vi "Template Test.vi"(0 "Limits File Path":path, 5 "Results File Path":path, 11 "error in":errorcluster) -> (15 "error out":errorcluster)   [LabVIEW 2024]
doc: "Template test"
uses:
  <vilib>/addons/_JKI Toolkits/State Machine/_JKI_lib_State_Machine.llb/Select State(s)_err__jki_lib_state_machine.vi
  <vilib>/addons/_JKI Toolkits/State Machine/_JKI_lib_State_Machine.llb/Periodic Trigger__ogtk__JKI-SM__jki_lib_state_machine.vi
  <userlib>/_OpenG.lib/file/file.llb/Strip Path Extension - String__ogtk.vi
  <vilib>/Utility/file.llb/Read Delimited Spreadsheet (string).vi
  <vilib>/Utility/file.llb/Write Delimited Spreadsheet (string).vi
  <userlib>/_OpenG.lib/file/file.llb/openg_file.lvlib
  <userlib>/_OpenG.lib/appcontrol/appcontrol.llb/openg_application_control.lvlib
  <userlib>/_OpenG.lib/time/time.llb/openg_time.lvlib
panel:
  out "Voltage Results Data":string[](array[string])
  in  "Exit":bool
  # "LED Test VI"
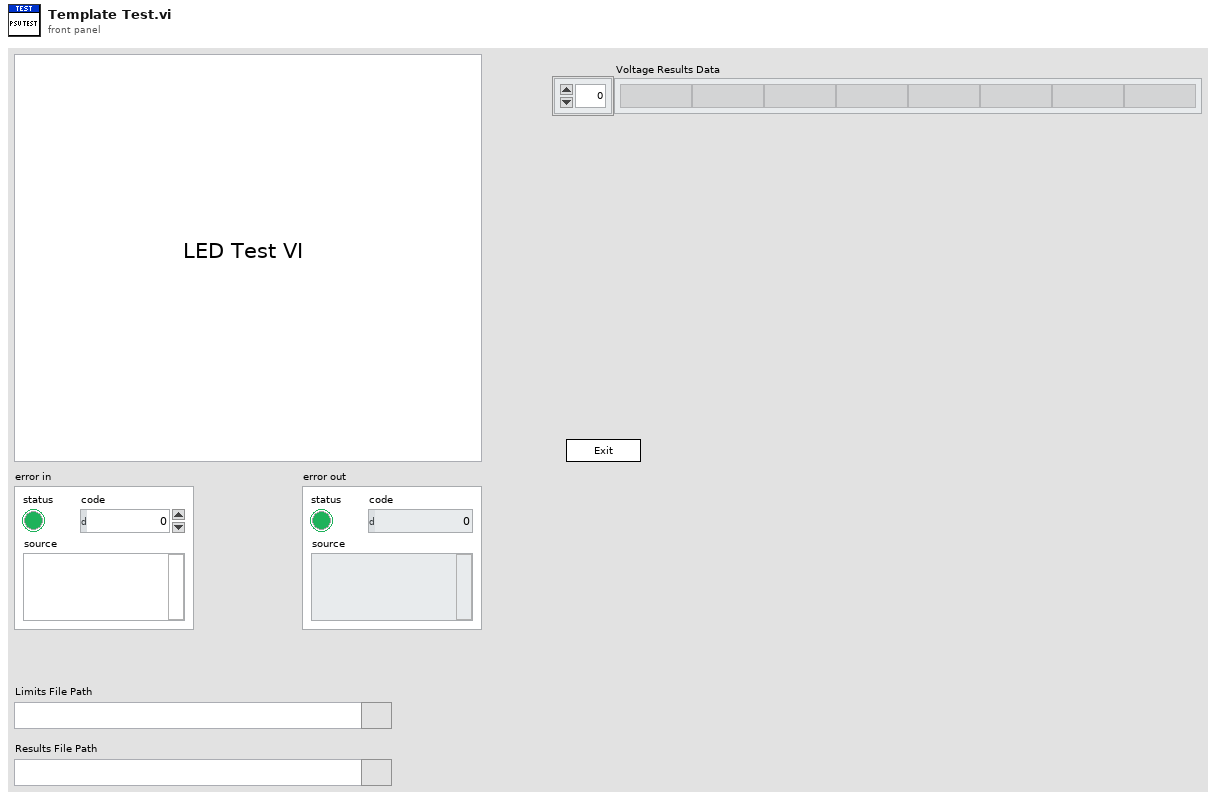
[diagram p1: front panel]
types:
  T1 = enum32{"Invalid", "Standard", "Closed", "Hidden", "Minimized", "Maximized"}
  T2 = enum32{"invalid app kind", "Development System", "Run Time System", "Student Edition", "Embedded LabVIEW", "Evaluation", "Custom"}
  T3 = cluster{"Core":cluster{"Current VI Reference":refnum<vi>, "Close Panel on Exit?":bool}, "Limits File Path":path, "Test Limits":string[][], "Results Data Array":string[][], "Results File Path":path, "Voltage":dbl}
  T4 = cluster{"Current VI Reference":refnum<vi>, "Close Panel on Exit?":bool}
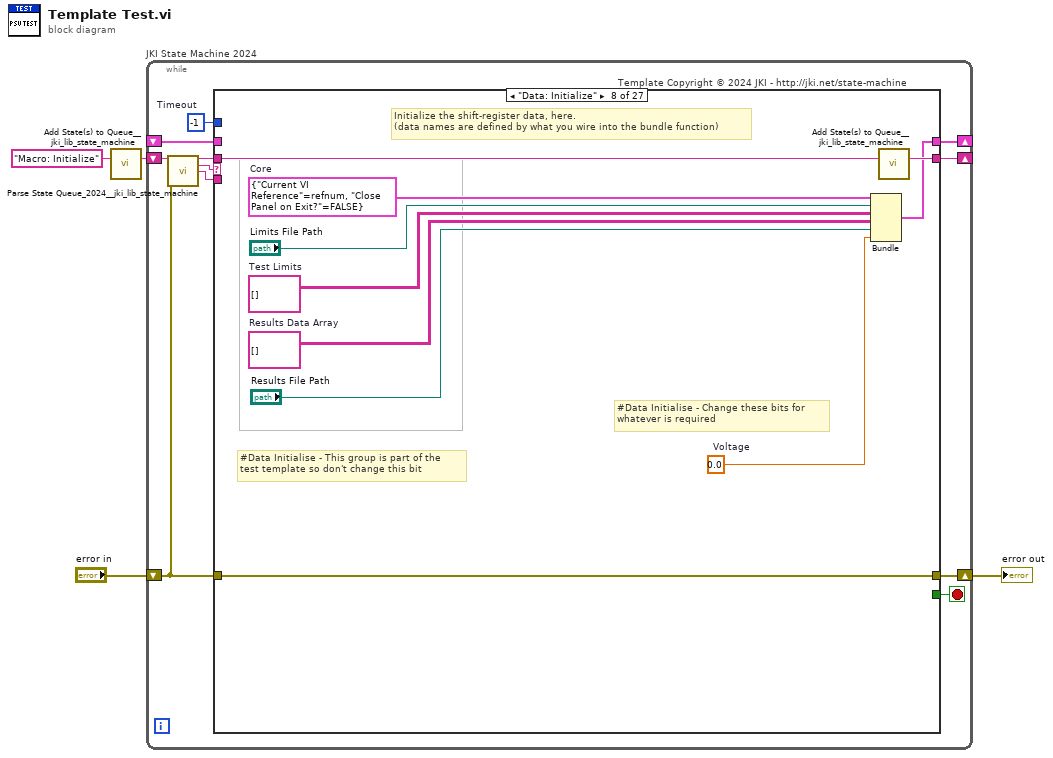
[diagram p0: block diagram]
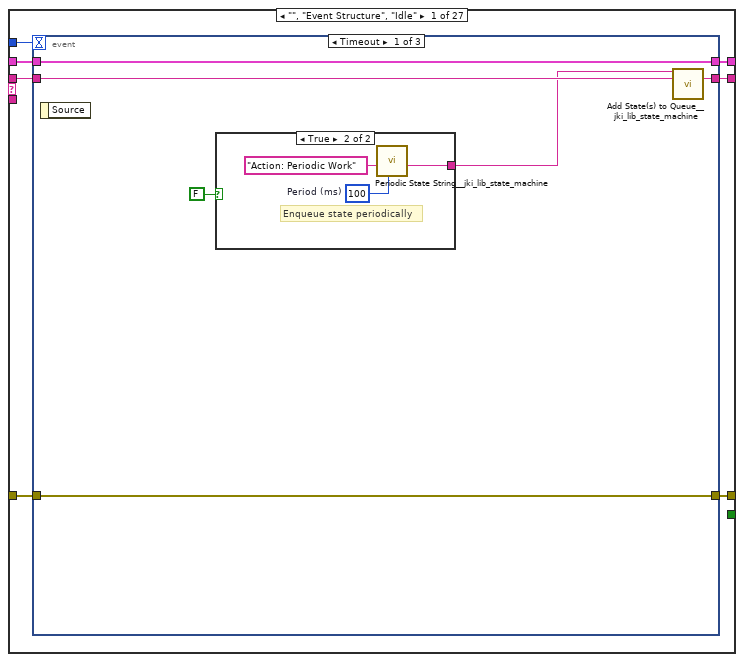
[diagram p2: hidden frame]
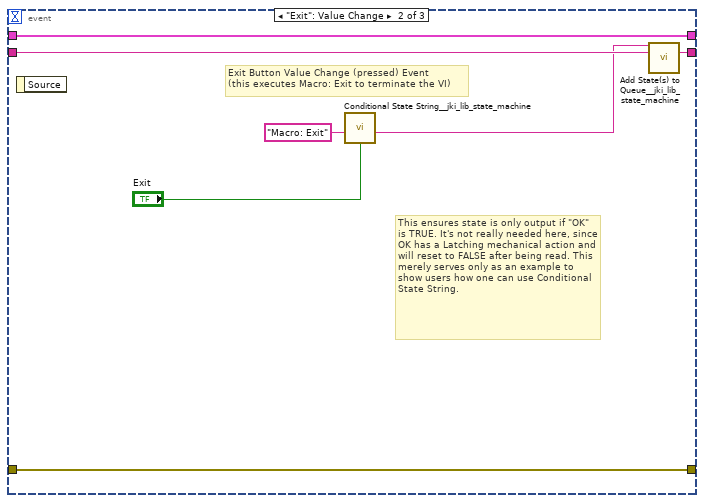
[diagram p4: hidden frame]
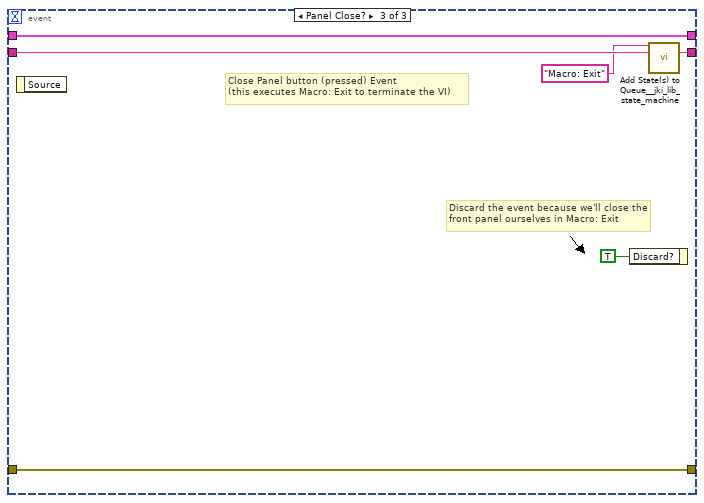
[diagram p5: hidden frame]
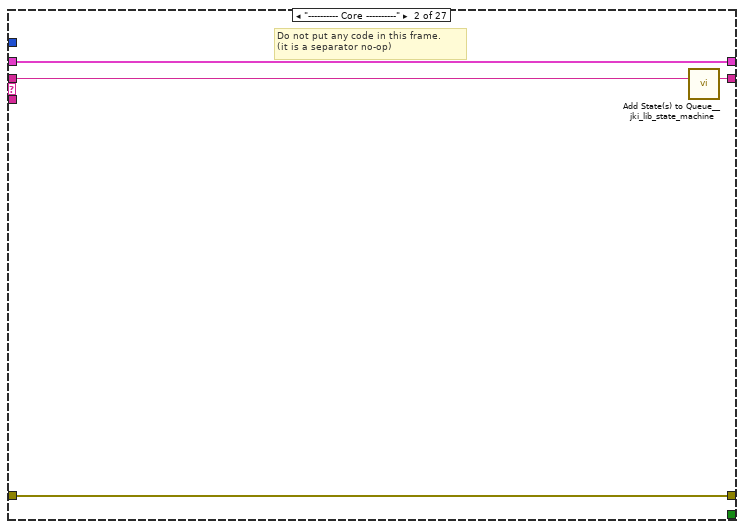
[diagram p6: hidden frame]
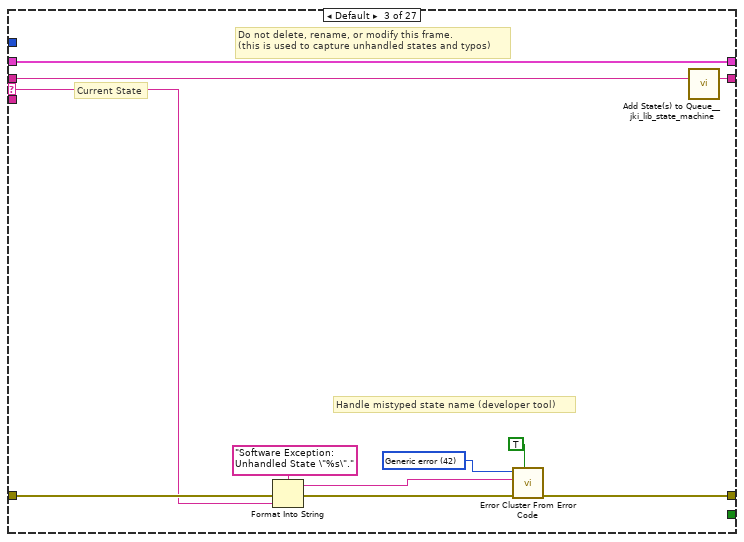
[diagram p7: hidden frame]
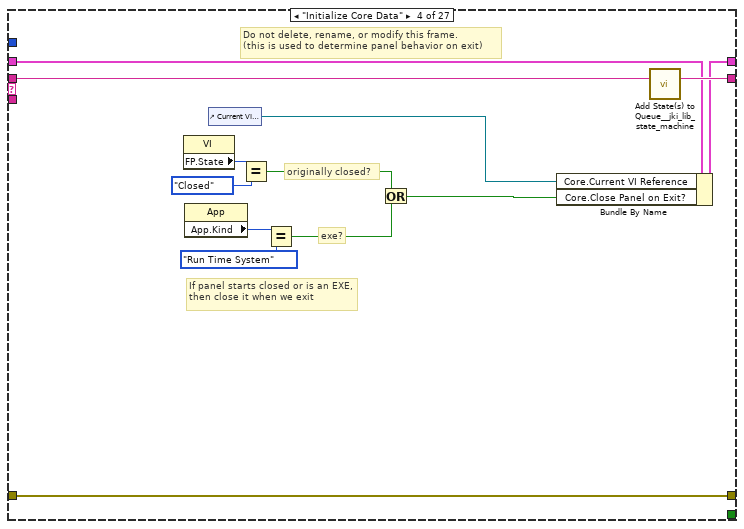
[diagram p8: hidden frame]
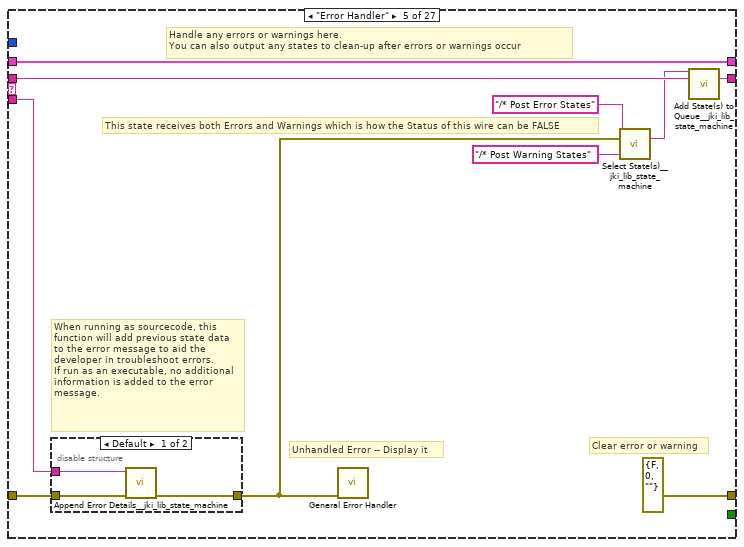
[diagram p9: hidden frame]
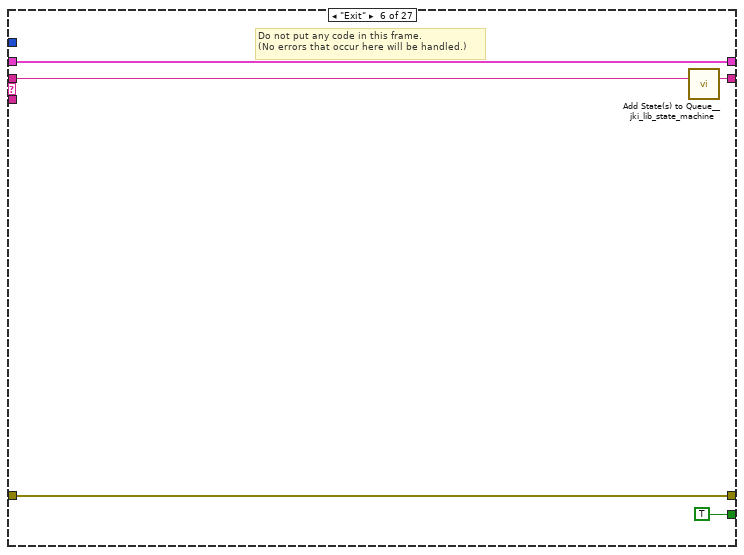
[diagram p11: hidden frame]
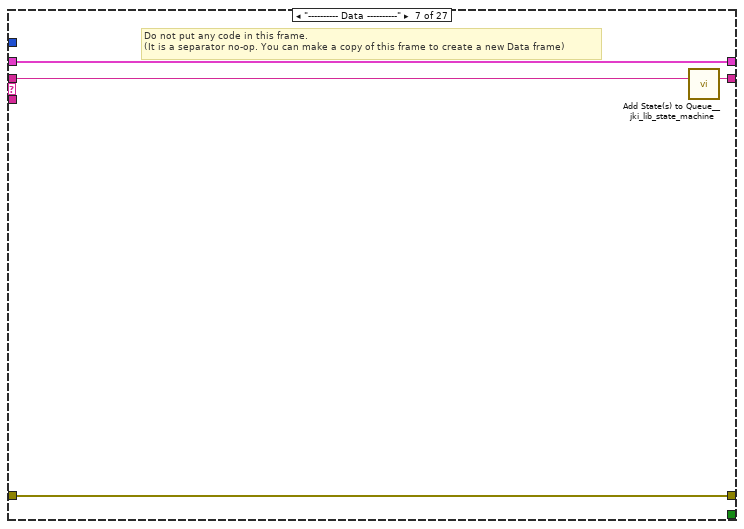
[diagram p12: hidden frame]
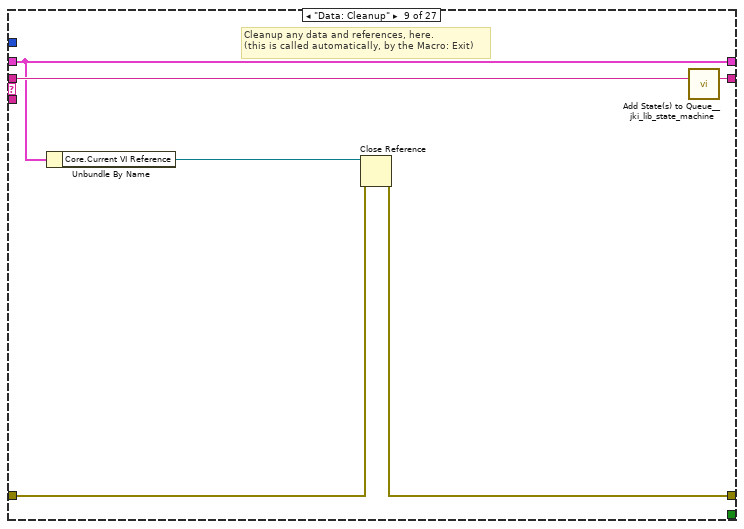
[diagram p13: hidden frame]
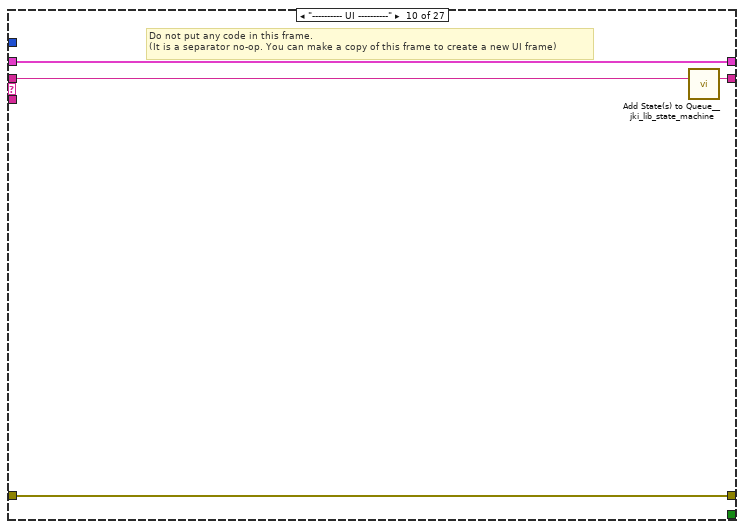
[diagram p14: hidden frame]
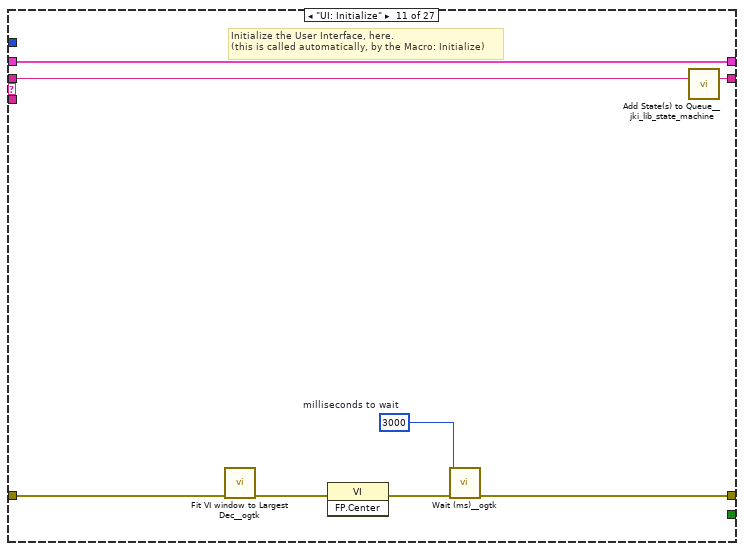
[diagram p15: hidden frame]
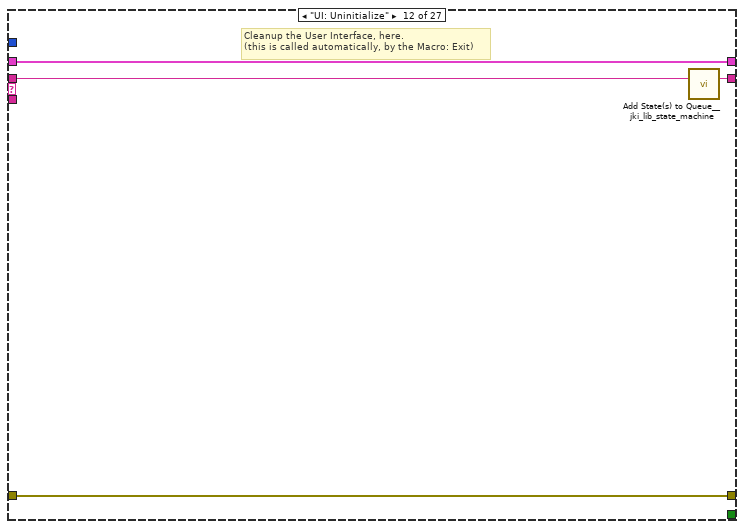
[diagram p16: hidden frame]
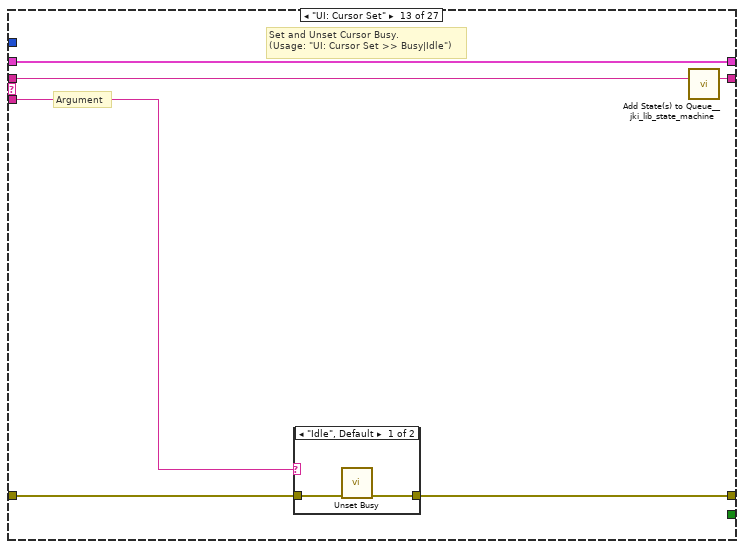
[diagram p17: hidden frame]
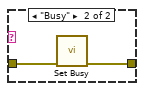
[diagram p18: hidden frame]
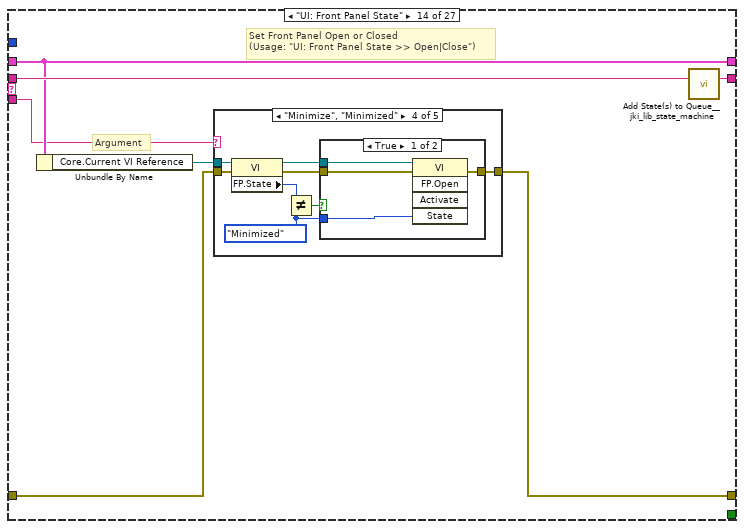
[diagram p19: hidden frame]
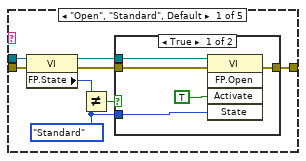
[diagram p20: hidden frame]
diagram:
  n1 = call <vilib>:"Add State(s) to Queue__jki_lib_state_machine.vi"("State(s) in (\"\")"="Macro: Initialize") -> ("States Out"=w4:string)  [unwired: 14 in]
  n2 = while "JKI State Machine 2024" {
    shift-right: [w8] -> _
    shift-left: _ -> [w7]
    shift-right: [w11] -> w1
    shift-left: "error in" -> [w5]
    shift-right: [w10] -> _
    shift-left: w4 -> [w12]
    stop <- w9 stop-if-true
    w6 = -1  # Timeout
    # "Template Copyright © 2024 JKI - http://jki.net/state-machine"
    n3 = call <vilib>:"Parse State Queue_2024__jki_lib_state_machine.vi"("State Queue"=w12, "Error In (no error)"=w5) -> ("Remaining States"=w14:string, "Current State"=w15:string, "Arguments"=w13:string)  [unwired: 11 in]
    n4 = case shown="\"Data: Initialize\"" w15 {
      selector: w15 -> [_ _ w49 _ _ _ _ _ _ _ _ _ _ _ _ _ _ _ _ _ _ _ _ _ _ _ _]
      tunnel: w14 -> [w22 w48 w53 w72 w82 w91 w95 w105 w111 w115 w123 w127 w133 w144 w213 w218 w222 w231 w235 w248 w265 w269 w278 w282 w286 w292 w296]
      tunnel: w13 -> [_ _ _ _ w77 _ _ _ _ _ _ _ w128 w138 _ _ _ _ _ _ _ _ _ _ _ _ _]
      tunnel: w7 -> [w20 w45 w51 w65 w79 w89 w92 _ w106 w112 w121 w125 w131 w140 w210 w215 w219 w229 w232 w238 w257 w266 w274 w279 w283 w289 w293]
      tunnel: [w19 w46 w55 w69 errorcluster {"status"=FALSE, "code"=0, "source"=""} ("error out") w88 w93 w102 w107 w113 w119 w124 w129 w141 w211 w216 w220 w226 w233 w244 w262 w267 w276 w280 w284 w290 w294] -> w11
      tunnel: w5 -> [w16 w46 w54 w69 w78 w88 w93 w102 w108 w113 w120 w124 w130 w142 w211 w216 w220 w226 w233 w243 w261 w267 w275 w280 w284 w290 w294]
      tunnel: [w21 w47 w52 w71 w81 w90 w94 w104 w110 w114 w122 w126 w132 w143 w212 w217 w221 w230 w234 w247 w264 w268 w277 w281 w285 w291 w295] -> w10
      tunnel: [_ _ _ _ _ TRUE _ _ _ _ _ _ _ _ _ _ _ _ _ _ _ _ _ _ _ _ _] -> w9
      tunnel: [w18 w45 w51 w70 w79 w89 w92 w103 w106 w112 w121 w125 w131 w140 w210 w215 w219 w229 w232 w237 w256 w266 w274 w279 w283 w288 w293] -> w8
      tunnel: w6 -> [w17 _ _ _ _ _ _ _ _ _ _ _ _ _ _ _ _ _ _ _ _ _ _ _ _ _ _]
      frame "", "Event Structure", "Idle" {
        n5 = event shown="[0] Timeout" {
          selector: _ -> [_ _ _]
          dyn-events: _ -> [_ _ _]
          timeout: w17 -> [_ _ _]
          tunnel: w22 -> [w28 w38 w44]
          tunnel: [w27 w37 w43] -> w21
          tunnel: w20 -> [w25 w35 w41]
          tunnel: [w26 w36 w42] -> w19
          tunnel: w16 -> [w26 w36 w42]
          tunnel: [w25 w35 w41] -> w18
          event Timeout {
            n6 = event-data() -> ()  [unwired: 1 in, 1 out]
            n7 = case shown="True" FALSE {
              tunnel: [_ w31] -> w24
              frame False {
              }
              frame True {
                w29 = u32 100  # Period (ms)
                # "Enqueue state periodically"
                n8 = call <vilib>:"Periodic State String__jki_lib_state_machine.vi"("Period (ms)"=w29, "State"="Action: Periodic Work") -> ("State Out"=w31:string)  [unwired: 9 in]
              }
            }
            n9 = call <vilib>:"Add State(s) to Queue__jki_lib_state_machine.vi"("State(s) in Front (\"\")"=w24, "State(s) in (\"\")"=w28) -> ("States Out"=w27:string)  [unwired: 13 in]
          }
          event "Exit": Value Change {
            # "This ensures state is only output if \"OK\" is TRUE. It's not really needed here, since OK has a Latching mechanical action and will reset to FALSE after being read. This merely serves only as an example to show users how one can use Conditional State String."
            # "Exit Button Value Change (pressed) Event\n(this executes Macro: Exit to terminate the VI)"
            n10 = event-data() -> ()  [unwired: 1 in, 1 out]
            n11 = call <vilib>:"Conditional State String__jki_lib_state_machine.vi"("Do State(s)?"="Exit", "State"="Macro: Exit") -> ("State Out"=w32:string)  [unwired: 7 in]
            n12 = call <vilib>:"Add State(s) to Queue__jki_lib_state_machine.vi"("State(s) in Front (\"\")"=w32, "State(s) in (\"\")"=w38) -> ("States Out"=w37:string)  [unwired: 13 in]
          }
          event Panel Close? {
            # "Discard the event because we'll close the front panel ourselves in Macro: Exit"
            # "Close Panel button (pressed) Event\n(this executes Macro: Exit to terminate the VI)"
            n13 = event-data() -> ()  [unwired: 1 in, 1 out]
            n14 = event-data("Discard?"=TRUE) -> ()  [unwired: 1 in, 1 out]
            n15 = call <vilib>:"Add State(s) to Queue__jki_lib_state_machine.vi"("State(s) in Front (\"\")"="Macro: Exit", "State(s) in (\"\")"=w44) -> ("States Out"=w43:string)  [unwired: 13 in]
          }
        }
      }
      frame "---------- Core ----------" {
        # "Do not put any code in this frame.\n(it is a separator no-op)"
        n16 = call <vilib>:"Add State(s) to Queue__jki_lib_state_machine.vi"("State(s) in (\"\")"=w48) -> ("States Out"=w47:string)  [unwired: 14 in]
      }
      frame Default {
        w58 = 42 items=["No error", "Argument error", "Memory is full", "Out of zone", "End of file", "File already open", "Generic file I/O error", "File not found", "File permission error", "Disk is full", "Duplicate path", "Too many files open", "System feature not enabled", "Resource file not found", "Cannot add resource", "Resource not found", "Image not found", "Image memory error", "Pen does not exist", "Config type invalid", "Config token not found", "Config parse error", "Config memory error", "Bad external code format", "Bad external code offset", "External code not present", "Null window", "Destroy window error", "Null menu", "Print aborted", "Bad print record", "Print driver error", "Windows error during printing", "Memory error during printing", "Print dialog error", "Generic print error", "Invalid device refnum", "Device not found", "Device parameter error", "Device unit error", "Cannot open device", "Device call aborted", "Generic error", "Cancelled by user", "Object ID too low", "Object ID too high", "Object not in heap", "Unknown heap", "Unknown object (invalid DefProc)", "Unknown object (DefProc not in table)", "Message out of range", "Invalid (null) method", "Unknown message", "Manager call not supported", "Bad address", "Network operation in progress", "Network operation timed out", "Connection is busy", "Network attribute not supported", "Network error", "Address in use", "System out of memory", "Connection aborted", "Connection refused", "Not connected", "Already connected", "Connection closed", "Initialization error (interapplication manager)", "Bad occurrence", "Wait on unbound occurrence handler", "Occurrence queue overflow", "Datalog type conflict", "Unused", "Unrecognized type (interapplication manager)", "Memory corrupt", "Failed to make temporary DLL", "Old CIN version", "Drag socket not found", "Failed to load drop-object", "Failed to register OLE object", "Failed to release OLE object", "Format specifier type mismatch", "Unknown format specifier", "Too few format specifiers", "Too many format specifiers", "Scan failed", "Newer CIN version", "Error converting to variant", "Runtime menu error", "Password tampered", "Variant attribute not found", "Incompatible variant data type", "Event data is not available", "Event Store is not present", "Occurrence is not found", "Event Queue is not created", "Event info is not available", "Refnum passed is NULL", "Error retrieving Class GUID", "Error retrieving CoClass GUID", "Error retrieving TypeLib GUID.", "Bad built application magic bytes.", "Specific driver is different from the specific driver associated with the Logical Name.", "There is no session opened to the class driver.", "Max Error", "MAX - Error with config objects", "MAX - Error loading configuration", "MAX - Group not supported"]
        # "Current State"
        # "Do not delete, rename, or modify this frame.\n(this is used to capture unhandled states and typos)"
        # "Handle mistyped state name (developer tool)"
        n17 = Format Into String(format string="Software Exception: Unhandled State \"%s\"." ("message"), error in=w54, w49) -> (resulting string=w57:string, error out=w56:errorcluster)  [unwired: 1 in]
        n18 = call <vilib>:"Error Cluster From Error Code.vi"("show call chain? (False)"=TRUE, "error in (no error)"=w56, "error message (\"\")"=w57, "error code (0)"=w58) -> ("error out"=w55:errorcluster)  [unwired: 5 in]
        n19 = call <vilib>:"Add State(s) to Queue__jki_lib_state_machine.vi"("State(s) in (\"\")"=w53) -> ("States Out"=w52:string)  [unwired: 14 in]
      }
      frame "Initialize Core Data" {
        # "Do not delete, rename, or modify this frame.\n(this is used to determine panel behavior on exit)"
        # "originally closed?"
        # "exe?"
        # "If panel starts closed or is an EXE, then close it when we exit"
        n20 = property class="VI"() -> ("FP.State"=w62:T1)  [unwired: 2 in, 2 out]
        n21 = property class="App"() -> ("App.Kind"=w68:T2)  [unwired: 2 in, 2 out]
        n22 = control-ref of="Current VI Reference"() -> (w63:refnum<vi>)
        n23 = Equal?(x=w62, y=T1."Closed" ("Front Panel Window:State")) -> (x = y?=w60:bool)
        n24 = Equal?(x=w68, y=T2."Run Time System" ("Application:Kind")) -> (x = y?=w66:bool)
        n25 = Or(x=w60, y=w66) -> (x .or. y?=w64:bool)
        n26 = Bundle By Name(cluster=w65, "Core.Current VI Reference"=w63, "Core.Close Panel on Exit?"=w64) -> (w70:T3)
        n27 = call <vilib>:"Add State(s) to Queue__jki_lib_state_machine.vi"("State(s) in (\"\")"=w72) -> ("States Out"=w71:string)  [unwired: 14 in]
      }
      frame "Error Handler" {
        # "When running as sourcecode, this function will add previous state data to the error message to aid the developer in troubleshoot errors.\nIf run as an executable, no additional information is added to the error message."
        # "This state receives both Errors and Warnings which is how the Status of this wire can be FALSE"
        # "Unhandled Error -- Display it"
        # "Handle any errors or warnings here.\nYou can also output any states to clean-up after errors or warnings occur"
        # "Clear error or warning"
        n28 = disable-structure shown="Default" {
          disable-tunnel: w78 -> [w85 w86]
          disable-tunnel: w77 -> [w84 _]
          disable-tunnel: [w83 w86] -> w76
          frame condition #0 (active) {
            n29 = call <vilib>:"Append Error Details__jki_lib_state_machine.vi"("error in (no error)"=w85, "Previous State and Argument(s)"=w84) -> ("error out"=w83:errorcluster)  [unwired: 9 in]
          }
          frame condition #1 {
          }
        }
        n30 = call <vilib>:"General Error Handler.vi"("error in (no error)"=w76) -> ()  [unwired: 10 in, 5 out]
        n31 = call-poly <vilib>:"Select State(s)__jki_lib_state_machine.vi"("State(s) if True (\"\")"="/* Post Error States", "Select"=w76, "State(s) if False (\"\")"="/* Post Warning States") -> ("States Out"=w74:string)  [unwired: 12 in]
        n32 = call <vilib>:"Add State(s) to Queue__jki_lib_state_machine.vi"("State(s) in Front (\"\")"=w74, "State(s) in (\"\")"=w82) -> ("States Out"=w81:string)  [unwired: 13 in]
      }
      frame "Exit" {
        # "Do not put any code in this frame.\n(No errors that occur here will be handled.)"
        n33 = call <vilib>:"Add State(s) to Queue__jki_lib_state_machine.vi"("State(s) in (\"\")"=w91) -> ("States Out"=w90:string)  [unwired: 14 in]
      }
      frame "---------- Data ----------" {
        # "Do not put any code in this frame.\n(It is a separator no-op. You can make a copy of this frame to create a new Data frame)"
        n34 = call <vilib>:"Add State(s) to Queue__jki_lib_state_machine.vi"("State(s) in (\"\")"=w95) -> ("States Out"=w94:string)  [unwired: 14 in]
      }
      frame "Data: Initialize" {
        w96 = 0.0  # Voltage
        w98 = string[][] []  # Results Data Array
        w99 = string[][] []  # Test Limits
        w101 = T4 {"Current VI Reference"=refnum, "Close Panel on Exit?"=FALSE}  # Core
        # "#Data Initialise - Change these bits for\nwhatever is required"
        # "#Data Initialise - This group is part of the\ntest template so don't change this bit"
        # "Initialize the shift-register data, here.\n(data names are defined by what you wire into the bundle function)"
        n35 = Bundle("Core"=w101, "Limits File Path"="Limits File Path", "Test Limits"=w99, "Results Data Array"=w98, "Results File Path"="Results File Path", "Voltage"=w96) -> (w103:T3)  [unwired: 1 in]
        n36 = call <vilib>:"Add State(s) to Queue__jki_lib_state_machine.vi"("State(s) in (\"\")"=w105) -> ("States Out"=w104:string)  [unwired: 14 in]
      }
      frame "Data: Cleanup" {
        # "Cleanup any data and references, here.\n(this is called automatically, by the Macro: Exit)"
        n37 = Unbundle By Name(w106) -> ("Core.Current VI Reference"=w109:refnum<vi>)
        n38 = Close Reference(reference=w109, error in (no error)=w108) -> (error out=w107:errorcluster)
        n39 = call <vilib>:"Add State(s) to Queue__jki_lib_state_machine.vi"("State(s) in (\"\")"=w111) -> ("States Out"=w110:string)  [unwired: 14 in]
      }
      frame "---------- UI ----------" {
        # "Do not put any code in this frame.\n(It is a separator no-op. You can make a copy of this frame to create a new UI frame)"
        n40 = call <vilib>:"Add State(s) to Queue__jki_lib_state_machine.vi"("State(s) in (\"\")"=w115) -> ("States Out"=w114:string)  [unwired: 14 in]
      }
      frame "UI: Initialize" {
        w118 = u32 3000  # milliseconds to wait
        # "Initialize the User Interface, here.\n(this is called automatically, by the Macro: Initialize)"
        n41 = call <userlib>:"Fit VI window to Largest Dec__ogtk.vi"("error in (no error)"=w120) -> ("error out"=w116:errorcluster)  [unwired: 5 in, 1 out]
        n42 = invoke class="VI" method="FP.Center"(error in=w116) -> (error out=w117:errorcluster)  [unwired: 2 in, 2 out]
        n43 = call <userlib>:"Wait (ms)__ogtk.vi"("error in (no error)"=w117, "milliseconds to wait"=w118) -> ("error out"=w119:errorcluster)  [unwired: 8 in, 1 out]
        n44 = call <vilib>:"Add State(s) to Queue__jki_lib_state_machine.vi"("State(s) in (\"\")"=w123) -> ("States Out"=w122:string)  [unwired: 14 in]
      }
      frame "UI: Uninitialize" {
        # "Cleanup the User Interface, here.\n(this is called automatically, by the Macro: Exit)"
        n45 = call <vilib>:"Add State(s) to Queue__jki_lib_state_machine.vi"("State(s) in (\"\")"=w127) -> ("States Out"=w126:string)  [unwired: 14 in]
      }
      frame "UI: Cursor Set" {
        # "Argument"
        # "Set and Unset Cursor Busy.\n(Usage: \"UI: Cursor Set >> Busy|Idle\")"
        n46 = case shown="\"Idle\", Default" w128 {
          tunnel: w130 -> [w135 w137]
          tunnel: [w134 w136] -> w129
          frame "Idle", Default {
            n47 = call <vilib>:"Unset Busy.vi"("error in (no error)"=w135) -> ("error out"=w134:errorcluster)  [unwired: 10 in]
          }
          frame "Busy" {
            n48 = call <vilib>:"Set Busy.vi"("error in (no error)"=w137) -> ("error out"=w136:errorcluster)  [unwired: 9 in, 1 out]
          }
        }
        n49 = call <vilib>:"Add State(s) to Queue__jki_lib_state_machine.vi"("State(s) in (\"\")"=w133) -> ("States Out"=w132:string)  [unwired: 14 in]
      }
      frame "UI: Front Panel State" {
        # "Argument"
        # "Set Front Panel Open or Closed\n(Usage: \"UI: Front Panel State >> Open|Close\")"
        n50 = Unbundle By Name(w140) -> ("Core.Current VI Reference"=w139:refnum<vi>)
        n51 = case shown="\"Minimize\", \"Minimized\"" w138 {
          tunnel: w142 -> [w150 w165 w176 w189 w202]
          tunnel: [w152 w166 w178 w191 w204] -> w141
          tunnel: w139 -> [w151 w163 w177 w190 w203]
          frame "Open", "Standard", Default {
            w145 = T1."Standard" ("State")
            n52 = property class="VI"(reference=w151, error in=w150) -> (reference out=w148:refnum<vi>, error out=w149:errorcluster, "FP.State"=w147:T1)
            n53 = Not Equal?(x=w147, y=w145) -> (x != y?=w146:bool)
            n54 = case shown="True" w146 {
              tunnel: [w156 w158] -> w152
              tunnel: w149 -> [w155 w158]
              tunnel: w148 -> [w154 _]
              tunnel: w145 -> [w153 _]
              frame True {
                n55 = invoke class="VI" method="FP.Open"(reference=w154, error in=w155, "Activate"=TRUE, "State"=w153) -> (error out=w156:errorcluster)  [unwired: 1 in, 4 out]
              }
              frame False {
              }
            }
          }
          frame "Close", "Closed" {
            n56 = property class="VI"(reference=w163, error in=w165) -> (reference out=w162:refnum<vi>, error out=w164:errorcluster, "FP.State"=w160:T1)
            n57 = Not Equal?(x=w160, y=T1."Closed" ("Front Panel Window:State")) -> (x != y?=w159:bool)
            n58 = case shown="True" w159 {
              tunnel: [w167 w170] -> w166
              tunnel: w164 -> [w167 w169]
              tunnel: w162 -> [_ w168]
              frame False {
              }
              frame True {
                n59 = invoke class="VI" method="FP.Close"(reference=w168, error in=w169) -> (error out=w170:errorcluster)  [unwired: 1 in, 2 out]
              }
            }
          }
          frame "Hidden", "Hide" {
            w171 = T1."Hidden" ("State")
            n60 = property class="VI"(reference=w177, error in=w176) -> (reference out=w174:refnum<vi>, error out=w175:errorcluster, "FP.State"=w173:T1)
            n61 = Not Equal?(x=w173, y=w171) -> (x != y?=w172:bool)
            n62 = case shown="True" w172 {
              tunnel: [w182 w183] -> w178
              tunnel: w175 -> [w181 w183]
              tunnel: w174 -> [w180 _]
              tunnel: w171 -> [w179 _]
              frame True {
                n63 = invoke class="VI" method="FP.Open"(reference=w180, error in=w181, "State"=w179) -> (error out=w182:errorcluster)  [unwired: 2 in, 4 out]
              }
              frame False {
              }
            }
          }
          frame "Minimize", "Minimized" {
            w184 = T1."Minimized" ("State")
            n64 = property class="VI"(reference=w190, error in=w189) -> (reference out=w187:refnum<vi>, error out=w188:errorcluster, "FP.State"=w186:T1)
            n65 = Not Equal?(x=w186, y=w184) -> (x != y?=w185:bool)
            n66 = case shown="True" w185 {
              tunnel: [w195 w196] -> w191
              tunnel: w188 -> [w194 w196]
              tunnel: w187 -> [w193 _]
              tunnel: w184 -> [w192 _]
              frame True {
                n67 = invoke class="VI" method="FP.Open"(reference=w193, error in=w194, "State"=w192) -> (error out=w195:errorcluster)  [unwired: 2 in, 4 out]
              }
              frame False {
              }
            }
          }
          frame "Maximize", "Maximized" {
            w197 = T1."Maximized" ("State")
            n68 = property class="VI"(reference=w203, error in=w202) -> (reference out=w200:refnum<vi>, error out=w201:errorcluster, "FP.State"=w199:T1)
            n69 = Not Equal?(x=w199, y=w197) -> (x != y?=w198:bool)
            n70 = case shown="True" w198 {
              tunnel: [w208 w209] -> w204
              tunnel: w201 -> [w207 w209]
              tunnel: w200 -> [w206 _]
              tunnel: w197 -> [w205 _]
              frame True {
                n71 = invoke class="VI" method="FP.Open"(reference=w206, error in=w207, "State"=w205) -> (error out=w208:errorcluster)  [unwired: 2 in, 4 out]
              }
              frame False {
              }
            }
          }
        }
        n72 = call <vilib>:"Add State(s) to Queue__jki_lib_state_machine.vi"("State(s) in (\"\")"=w144) -> ("States Out"=w143:string)  [unwired: 14 in]
      }
      frame "---------- Macro ----------" {
        # "Do not put any code in this frame.\n(It is a separator no-op. You can make a copy of this frame to create a new Macro frame)"
        n73 = call <vilib>:"Add State(s) to Queue__jki_lib_state_machine.vi"("State(s) in (\"\")"=w213) -> ("States Out"=w212:string)  [unwired: 14 in]
      }
      frame "Macro: Initialize" {
        # "Initialization Macro\n(This is called once, when the VI starts)"
        n74 = call <vilib>:"Add State(s) to Queue__jki_lib_state_machine.vi"("State(s) in Front (\"\")"="Data: Initialize\nInitialize Core Data\nUI: Initialize\nUI: Front Panel State >> Open\nTemplate: Initialise\nMacro: Test", "State(s) in (\"\")"=w218) -> ("States Out"=w217:string)  [unwired: 13 in]
      }
      frame "Macro: Test" {
        (unwired) "Limits Test: Read Limits File\nTemplate: Measurment\nLimits Test: **Template Test**\nResults Data: Write Results Data\nMacro: Exit"  # Limits Test: Read Limits File Template: Measurment Limits Test: **Template Test** Results Data: Write Results Data Macro: Exit
        # "#Test Macro - Add the sequence \nfor measurments and limits testing here"
        n75 = call <vilib>:"Add State(s) to Queue__jki_lib_state_machine.vi"("State(s) in (\"\")"=w222) -> ("States Out"=w221:string)  [unwired: 14 in]
      }
      frame "Macro: Exit" {
        # "Exit Macro\n(This is called once, when the VI exits)"
        n76 = Unbundle By Name(w229) -> ("Core.Close Panel on Exit?"=w224:bool)
        n77 = call <vilib>:"Conditional State String__jki_lib_state_machine.vi"("Do State(s)?"=w224, "State"="UI: Front Panel State >> Close") -> ("State Out"=w223:string)  [unwired: 7 in]
        n78 = call <vilib>:"Add State(s) to Queue__jki_lib_state_machine.vi"("State(s) in (\"\")"=w223, "State(s) at Back (\"\")"="Template: Cleanup\nUI: Uninitialize\nData: Cleanup\nExit") -> ("States Out"=w227:string)  [unwired: 13 in]
        n79 = call <vilib>:"Add State(s) to Queue__jki_lib_state_machine.vi"("State(s) in Front (\"\")"=w227, "State(s) in (\"\")"=w231) -> ("States Out"=w230:string)  [unwired: 13 in]
      }
      frame "---------- Limits Test ----------" {
        # "Template Separator\n(You can make a copy of, or modify, this frame)"
        n80 = call <vilib>:"Add State(s) to Queue__jki_lib_state_machine.vi"("State(s) in (\"\")"=w235) -> ("States Out"=w234:string)  [unwired: 14 in]
      }
      frame "Limits Test: Read Limits File" {
        w241 = ","  # delimiter (\t)
        n81 = Unbundle By Name(w238) -> ("Limits File Path"=w242:path)
        n82 = Current VI's Path "Test Case Path"() -> (path=w246:path)
        n83 = call-poly <vilib>:"Read Delimited Spreadsheet.vi"("file path (dialog if empty)"=w242, "error in (no error)"=w243, "delimiter (\\t)"=w241) -> ("all rows"=w239:string[][], "error out"=w244:errorcluster)  [unwired: 7 in, 4 out]
        n84 = Strip Path(path=w246) -> (name=w245:string)  [unwired: 1 out]
        n85 = call-poly <userlib>:"Strip Path Extension__ogtk.vi"("path"=w245) -> ("root"=w240:string)  [unwired: 1 out]
        n86 = for {
          tunnel: w240 -> [w252]
          tunnel: w239 -> [w250] mode=indexing
          tunnel: [w250] -> w236 mode=indexing if=w249
          n87 = Index Array(array=w250) -> (element=w251:string)  [unwired: 1 in]
          n88 = Equal?(x=w252, y=w251) -> (x = y?=w249:bool)
        }
        n89 = Bundle By Name(cluster=w238, "Test Limits"=w236) -> (w237:T3)
        n90 = call <vilib>:"Add State(s) to Queue__jki_lib_state_machine.vi"("State(s) in (\"\")"=w248) -> ("States Out"=w247:string)  [unwired: 14 in]
      }
      frame "Limits Test: **Template Test**" {
        w258 = "**Sub Test Name**"  # Sub Test Name
        # "#Limits Testing - Add the sub test name for\ntest included in limits file"
        n91 = Unbundle By Name(w257) -> ("Results Data Array"=w255:string[][])
        n92 = Unbundle By Name(w257) -> ("Test Limits"=w259:string[][], "Voltage"=w263:dbl)
        n93 = To Variant(anything=w263) -> (Variant=w260:variant)
        n94 = call "Process Results.vi"("error in (no error)"=w261, "Measurment"=w260, "Test Limits"=w259, "Sub Test Name"=w258) -> ("error out"=w262:errorcluster, "Results Data"=w254:string[])  [unwired: 6 in]
        "Voltage Results Data" <- w254
        n95 = Build Array (concatenate)(w255, w254) -> (w253:string[][])
        n96 = Bundle By Name(cluster=w257, "Results Data Array"=w253) -> (w256:T3)
        n97 = call <vilib>:"Add State(s) to Queue__jki_lib_state_machine.vi"("State(s) in (\"\")"=w265) -> ("States Out"=w264:string)  [unwired: 14 in]
      }
      frame "---------- Results Data ----------" {
        # "Template Separator\n(You can make a copy of, or modify, this frame)"
        n98 = call <vilib>:"Add State(s) to Queue__jki_lib_state_machine.vi"("State(s) in (\"\")"=w269) -> ("States Out"=w268:string)  [unwired: 14 in]
      }
      frame "Results Data: Write Results Data" {
        w270 = ","  # delimiter (\t)
        w271 = TRUE  # append to file? (new file:F)
        n99 = Unbundle By Name(w274) -> ("Results File Path"=w273:path, "Results Data Array"=w272:string[][])
        n100 = call-poly <vilib>:"Write Delimited Spreadsheet.vi"("file path (dialog if empty)"=w273, "2D data"=w272, "append to file? (new file:F)"=w271, "error in (no error)"=w275, "delimiter (\\t)"=w270) -> ("error out"=w276:errorcluster)  [unwired: 9 in, 1 out]
        n101 = call <vilib>:"Add State(s) to Queue__jki_lib_state_machine.vi"("State(s) in (\"\")"=w278) -> ("States Out"=w277:string)  [unwired: 14 in]
      }
      frame "---------- Template ----------" {
        # "Template Separator\n(You can make a copy of, or modify, this frame)"
        n102 = call <vilib>:"Add State(s) to Queue__jki_lib_state_machine.vi"("State(s) in (\"\")"=w282) -> ("States Out"=w281:string)  [unwired: 14 in]
      }
      frame "Template: Initialise" {
        # "Measurement initialisation code goes here"
        n103 = call <vilib>:"Add State(s) to Queue__jki_lib_state_machine.vi"("State(s) in (\"\")"=w286) -> ("States Out"=w285:string)  [unwired: 14 in]
      }
      frame "Template: Measurment" {
        w287 = 12.0  # Voltage (V)
        # "Measurment Code here"
        n104 = Bundle By Name(cluster=w289, "Voltage"=w287) -> (w288:T3)
        n105 = call <vilib>:"Add State(s) to Queue__jki_lib_state_machine.vi"("State(s) in (\"\")"=w292) -> ("States Out"=w291:string)  [unwired: 14 in]
      }
      frame "Template: Cleanup" {
        # "Measurment cleanup code goes here"
        n106 = call <vilib>:"Add State(s) to Queue__jki_lib_state_machine.vi"("State(s) in (\"\")"=w296) -> ("States Out"=w295:string)  [unwired: 14 in]
      }
    }
  }
  "error out" <- w1
